vi "Transition Measurements N chan.vi"(6 "percent level settings":T4={"method"=enum."auto select", "histogram size"=256, "histogram method"=enum."mode", "reserved"=1.0} {"reserved" format="%0.2f"}, 7 "edge number (1)":i32=1 min=1, 8 "error in (no error)":errorcluster, 9 "reference levels":T3={"high ref level"=90.0, "mid ref level"=50.0, "low ref level"=10.0, "ref units"=1} {"ref units" items=["absolute", "percent"]; "high ref level" format="%.2p"; "low ref level" format="%.2p"; "mid ref level" format="%.2p"}, 10 "polarity (rising)":u16(ring)=1 items=["falling", "rising"], 11 "signal(s) in":waveform(dbl)[](array[waveform])) -> (0 "error out":errorcluster, 1 "post-transition":T2(array[cluster]), 2 "pre-transition":T2(array[cluster]), 3 "transition duration":dbl[](array[numeric]) format="%.2p", 4 "measurement info":T1(array[cluster]), 5 "slope":dbl[](array[numeric]) format="%.2p")   [LabVIEW 2020, in "NI_MAPro.lvlib"]
doc: "Accepts an input signal of a single waveform or an array of waveforms and measures the transition duration (rise or fall time), slew rate, undershoot, and overshoot of a selected positive or negative transition in each waveform. Wire data to the <B>signal in</B> input to determine the polymorphic instance to use or manually select the instance."
uses:
  NI_MAPro.lvlib
  NI_MABase.lvlib
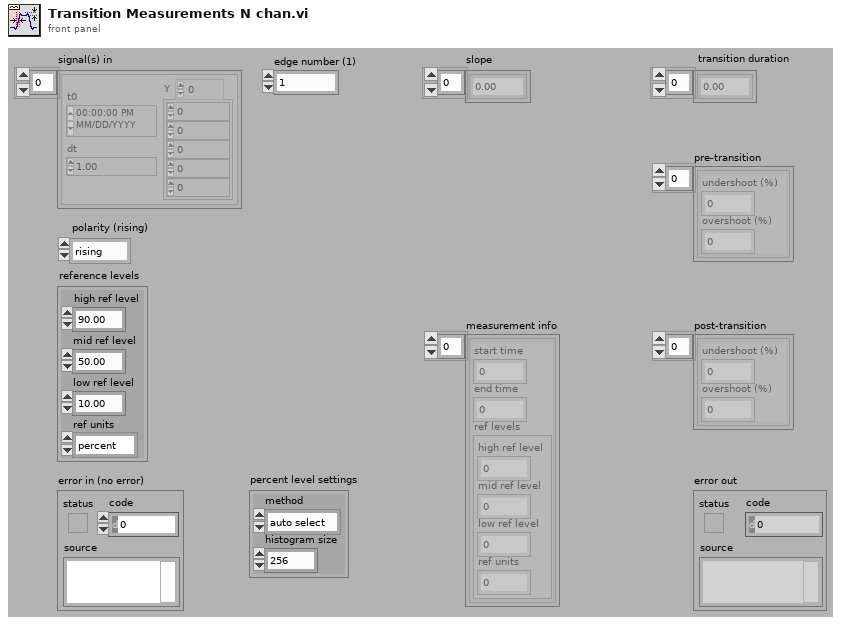
[diagram p1: front panel]
types:
  T1 = cluster{"start time":dbl, "end time":dbl, "ref levels":cluster{"high ref level":dbl, "mid ref level":dbl, "low ref level":dbl, "ref units":u16}}[]
  T2 = cluster{"undershoot (%)":dbl, "overshoot (%)":dbl}[]
  T3 = cluster{"high ref level":dbl, "mid ref level":dbl, "low ref level":dbl, "ref units":u16}
  T4 = cluster{"method":enum32{"histogram", "peak", "auto select"}, "histogram size":i32, "histogram method":enum16{"mode"}, "reserved":dbl}
  T5 = cluster{"undershoot (%)":dbl, "overshoot (%)":dbl}
  T6 = cluster{"start time":dbl, "end time":dbl, "ref levels":cluster{"high ref level":dbl, "mid ref level":dbl, "low ref level":dbl, "ref units":u16}}
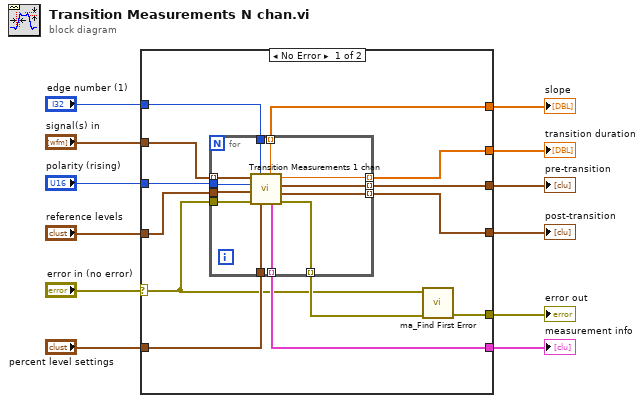
[diagram p0: block diagram]
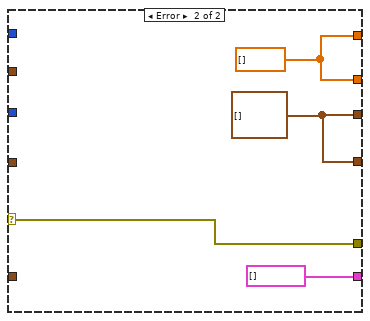
[diagram p2: hidden frame]
diagram:
  n1 = case shown="No Error" "error in (no error)" {
    selector: "error in (no error)" -> [w17 w41]
    tunnel: "percent level settings" -> [w24 _]
    tunnel: [w22 w41] -> w10
    tunnel: "signal(s) in" -> [w25 _]
    tunnel: "reference levels" -> [w21 _]
    tunnel: "edge number (1)" -> [w20 _]
    tunnel: "polarity (rising)" -> [w19 _]
    tunnel: [w16 w39] -> w5
    tunnel: [w18 T1 []] -> w1
    tunnel: [w15 w39] -> w4
    tunnel: [w14 w38] -> w3
    tunnel: [w13 w38] -> w2
    frame No Error {
      n2 = for {
        tunnel: w17 -> [w32]
        tunnel: w24 -> [w37]
        tunnel: [w36] -> w23 mode=indexing
        tunnel: w25 -> [w35] mode=indexing
        tunnel: w21 -> [w29]
        tunnel: w20 -> [w34]
        tunnel: w19 -> [w33]
        tunnel: [w31] -> w18 mode=indexing
        tunnel: [w30] -> w16 mode=indexing
        tunnel: [w28] -> w15 mode=indexing
        tunnel: [w27] -> w14 mode=indexing
        tunnel: [w26] -> w13 mode=indexing
        n3 = call "Transition Measurements 1 chan.vi"("percent level settings"=w37, "edge number (1)"=w34, "error in (no error)"=w32, "reference levels"=w29, "polarity (rising)"=w33, "signal in"=w35) -> ("error out"=w36:errorcluster, "post-transition"=w26:T5, "pre-transition"=w27:T5, "transition duration"=w28:dbl, "measurement info"=w31:T6, "slope"=w30:dbl)
      }
      n4 = call "ma_Find First Error.vi"("error array in"=w23, "error in 1 (no error)"=w17) -> ("error out"=w22:errorcluster)  [unwired: 2 in, 3 out]
    }
    frame Error {
      w38 = T2 []
      w39 = dbl[] []
    }
  }
  "error out" <- w10
  "transition duration" <- w4
  "slope" <- w5
  "pre-transition" <- w3
  "post-transition" <- w2
  "measurement info" <- w1
